vi "micro1 pvgen300.vi"(0 "FluxStrIn":string, 1 "Numin":i32, 5 "errin":errorcluster, 6 "Data label":string, 8 "tab ref":string[][](array[string]), 10 "ligne à traiter":string[](array[string])) -> (14 "result string":string, 15 "Numout":i32, 19 "errout":errorcluster)   [LabVIEW 2020]
uses:
  VG/VG_DeltaTcell.vi
  ZEN8 Semi Auto EMC/OP700/VG/VG_TCellmax.vi
  ZEN8 Semi Auto EMC/OP700/VG/VG_TCellmin.vi
  VG/IS30%.vi
  VG/VG_VCellMin70.vi
  VG/VG_VCellMax70.vi
  VG/VG_VCellMin30.vi
  VG/VG_VCellMax30.vi
  VG/VG_DeltaVcell.vi
  <vilib>/regexp/Match Regular Expression.xnode
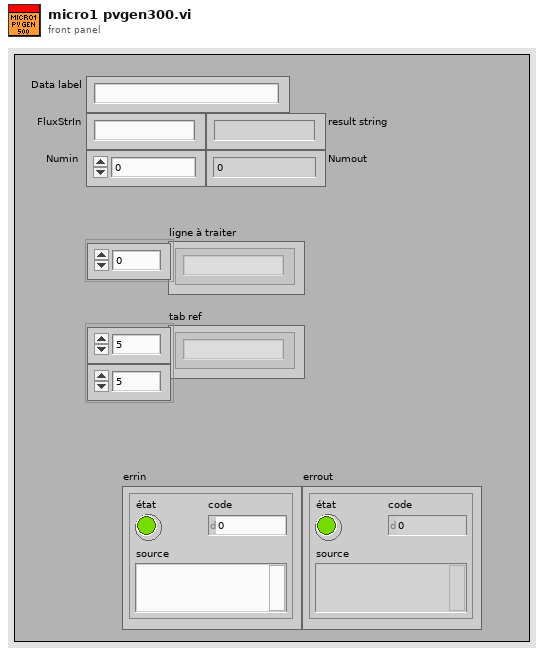
[diagram p1: front panel]
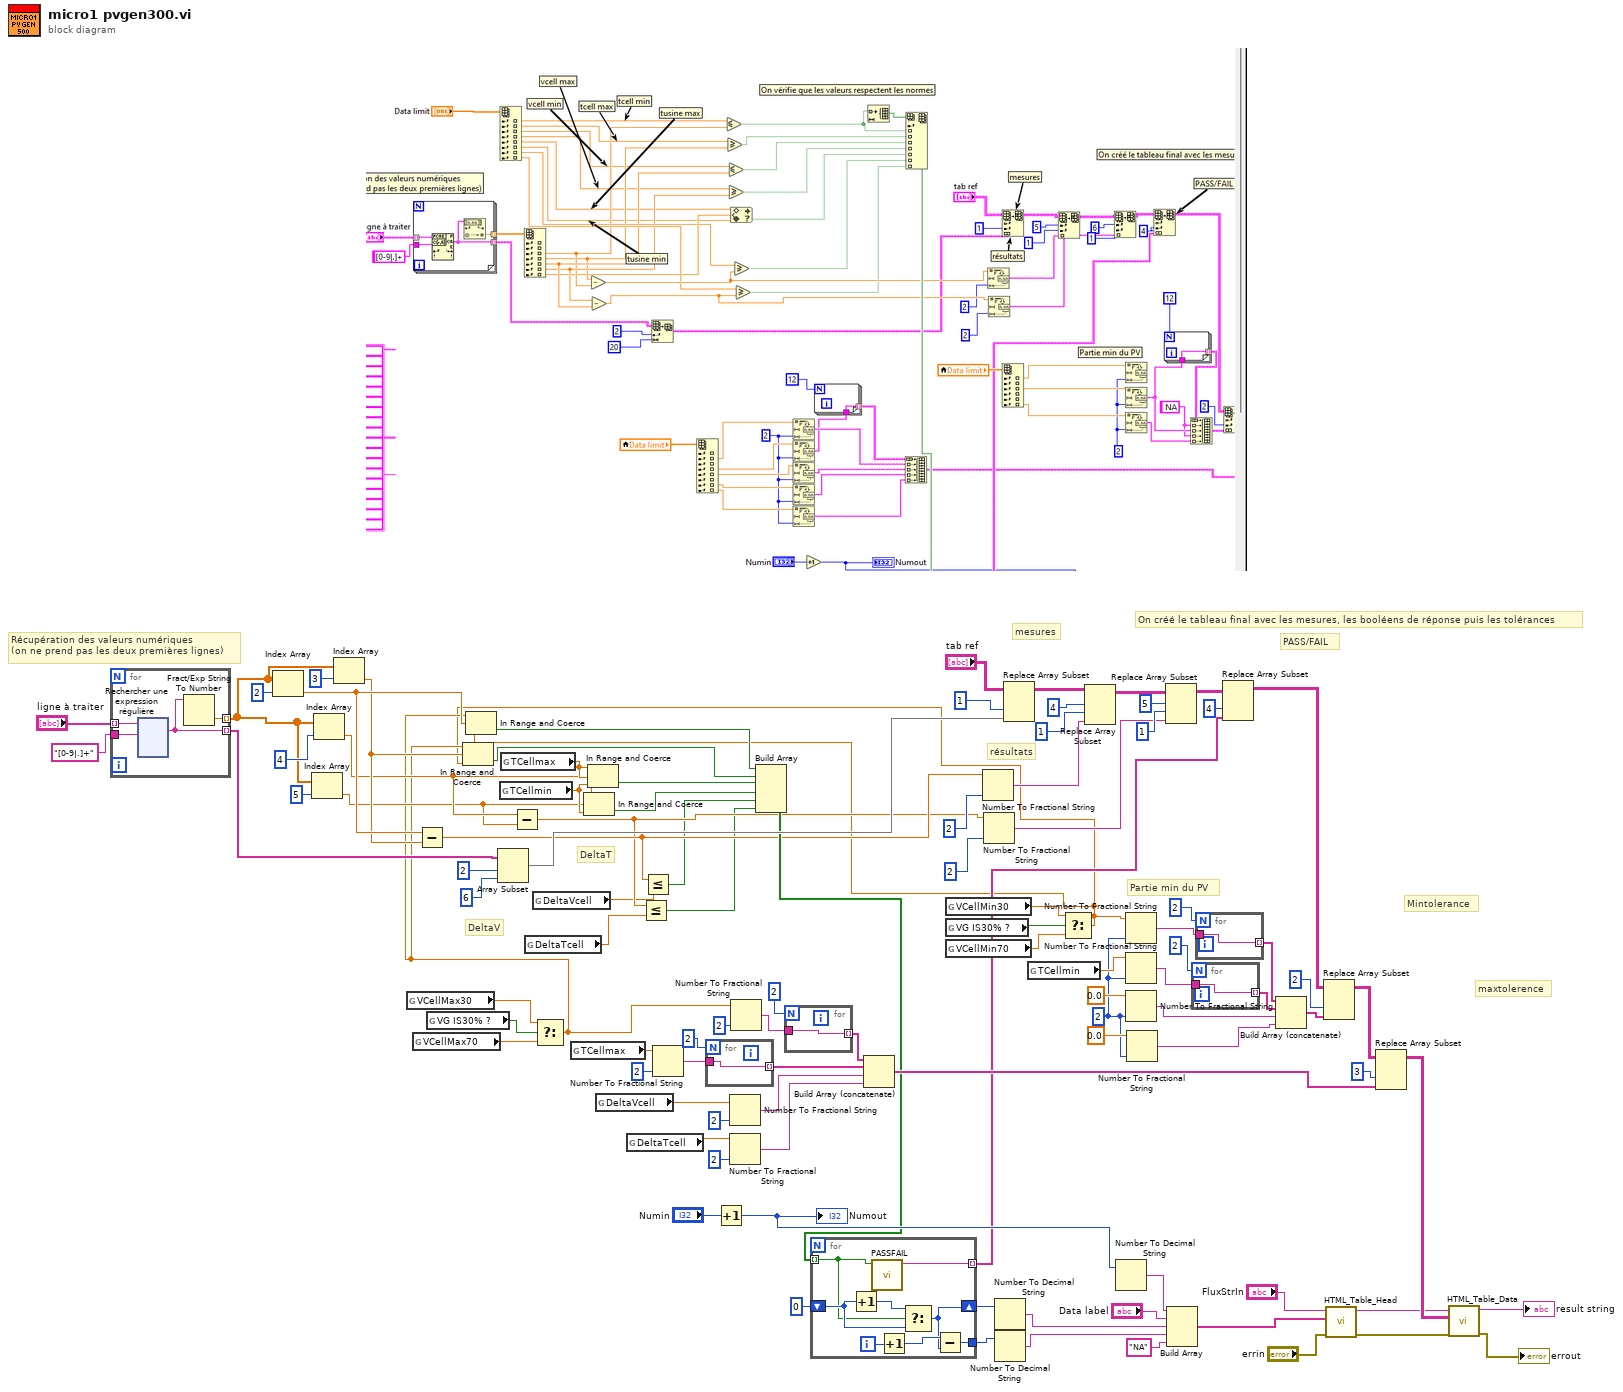
[diagram p0: block diagram]
diagram:
  w30 = 2
  # "DeltaV"
  # "DeltaT"
  # "Partie min du PV"
  # "Récupération des valeurs numériques\n(on ne prend pas les deux premières lignes)"
  # "On créé le tableau final avec les mesures, les booléens de réponse puis les tolérances"
  # "maxtolerence"
  # "Mintolerance"
  # "mesures"
  # "PASS/FAIL"
  # "résultats"
  n1 = for {
    tunnel: "ligne à traiter" -> [w106] mode=indexing
    tunnel: "[0-9|.]+" ("expression régulière") -> [w105]
    tunnel: [w104] -> w19 mode=indexing
    tunnel: [w103] -> w70 mode=indexing
    n2 = xnode "Rechercher une expression régulière"("input string"=w106, "regular expression"=w105) -> ("whole match"=w103:string)  [unwired: 4 in, 4 out]
    n3 = Fract/Exp String To Number(string=w103) -> (number=w104:dbl)  [unwired: 3 in, 1 out]
  }
  n4 = Index Array(array=w19, index=2 ("indice")) -> (element=w14:dbl)
  n5 = Index Array(array=w19, index=5 ("indice")) -> (element=w11:dbl)
  n6 = Index Array(array=w19, index=4 ("longueur")) -> (element=w12:dbl)
  n7 = Index Array(array=w19, index=3 ("indice")) -> (element=w13:dbl)
  n8 = global read "VG_VCellMax30.vi" "VCellMax30"() -> (w9:dbl)
  n9 = global read "VG_VCellMax70.vi" "VCellMax70"() -> (w8:dbl)
  n10 = Subtract(x=w14, y=w13) -> (x-y=w28:dbl)
  n11 = global read "IS30%.vi" "VG IS30% ?"() -> (w10:bool)
  n12 = Array Subset(array=w70, index=2 ("indice"), length=6 ("longueur")) -> (w73:string[])
  n13 = global read "VG_TCellmin.vi" "TCellmin"() -> (w16:dbl)
  n14 = global read "VG_TCellmax.vi" "TCellmax"() -> (w17:dbl)
  n15 = Subtract(x=w12, y=w11) -> (x-y=w26:dbl)
  n16 = global read "VG_DeltaTcell.vi" "DeltaTcell"() -> (w27:dbl)
  n17 = global read "VG_DeltaVcell.vi" "DeltaVcell"() -> (w2:dbl)
  n18 = Select(t=w9, s=w10, f=w8) -> (s? t:f=w4:dbl)
  n19 = global read "VG_TCellmax.vi" "TCellmax"() -> (w47:dbl)
  n20 = In Range and Coerce(upper limit=w17, x=w11, lower limit=w16) -> (In Range?=w15:bool)  [unwired: 1 out]
  n21 = In Range and Coerce(upper limit=w17, x=w12, lower limit=w16) -> (In Range?=w35:bool)  [unwired: 1 out]
  n22 = global read "VG_DeltaVcell.vi" "DeltaVcell"() -> (w1:dbl)
  n23 = global read "VG_DeltaTcell.vi" "DeltaTcell"() -> (w46:dbl)
  n24 = Less Or Equal?(x=w26, y=w27) -> (x <= y?=w25:bool)
  n25 = Less Or Equal?(x=w28, y=w2) -> (x <= y?=w23:bool)
  n26 = Number To Fractional String(number=w47, precision (6)=i16 2 ("précision (6)")) -> (F-format string=w43:string)  [unwired: 2 in]
  n27 = for {
    N: 2 -> [_]
    tunnel: w43 -> [w221]
    tunnel: [w221] -> w42 mode=indexing
  }
  n28 = Increment(x="Numin") -> (x+1=w88:i32)
  "Numout" <- w88
  n29 = Number To Fractional String(number=w1, precision (6)=i16 2 ("précision (6)")) -> (F-format string=w45:string)  [unwired: 2 in]
  n30 = Number To Fractional String(number=w46, precision (6)=i16 2 ("précision (6)")) -> (F-format string=w44:string)  [unwired: 2 in]
  n31 = Number To Fractional String(number=w4, precision (6)=i16 2 ("précision (6)")) -> (F-format string=w48:string)  [unwired: 2 in]
  n32 = for {
    N: 2 -> [_]
    tunnel: w48 -> [w222]
    tunnel: [w222] -> w57 mode=indexing
  }
  n33 = Build Array (concatenate)(w57, w42, w45, w44) -> (w102:string[])
  n34 = global read "VG_VCellMin30.vi" "VCellMin30"() -> (w5:dbl)
  n35 = global read "IS30%.vi" "VG IS30% ?"() -> (w7:bool)
  n36 = global read "VG_VCellMin70.vi" "VCellMin70"() -> (w6:dbl)
  n37 = Number To Fractional String(number=w28, precision (6)=i16 2) -> (F-format string=w62:string)  [unwired: 2 in]
  n38 = Number To Fractional String(number=w26, precision (6)=i16 2) -> (F-format string=w59:string)  [unwired: 2 in]
  n39 = Replace Array Subset(array="tab ref", new element=w73, index (col)=1 ("indice désactivé (col)")) -> (w66:string[][])  [unwired: 1 in]
  n40 = global read "VG_TCellmin.vi" "TCellmin"() -> (w40:dbl)
  n41 = Select(t=w5, s=w7, f=w6) -> (s? t:f=w3:dbl)
  n42 = In Range and Coerce(upper limit=w4, x=w13, lower limit=w3) -> (In Range?=w20:bool)  [unwired: 1 out]
  n43 = In Range and Coerce(upper limit=w4, x=w14, lower limit=w3) -> (In Range?=w22:bool)  [unwired: 1 out]
  n44 = Build Array(w22, w20, w35, w15, w23, w25) -> (w34:bool[])
  n45 = for {
    tunnel: w34 -> [w223] mode=indexing
    tunnel: [w224] -> w71 mode=indexing
    shift-right: [w226] -> w90
    shift-left: 0 -> [w229]
    tunnel: [w225] -> w91
    i -> [w228]
    n46 = Increment(x=w229) -> (x+1=w230:i32)
    n47 = call <userlib>:"PASSFAIL.vi"("E"=w223) -> ("S"=w224:string)  [unwired: 10 in]
    n48 = Increment(x=w228) -> (x+1=w227:i32)
    n49 = Select(t=w230, s=w223, f=w229) -> (s? t:f=w226:i32)
    n50 = Subtract(x=w227, y=w226) -> (x-y=w225:i32)
  }
  n51 = Number To Decimal String(number=w90) -> (decimal integer string=w92:string)  [unwired: 1 in]
  n52 = Number To Decimal String(number=w91) -> (decimal integer string=w93:string)  [unwired: 1 in]
  n53 = Replace Array Subset(array=w66, new element=w62, index (row)=4 ("disabled index (row)"), index (col)=1 ("disabled index (col)")) -> (w64:string[][])
  n54 = Number To Decimal String(number=w88) -> (decimal integer string=w76:string)  [unwired: 1 in]
  n55 = Number To Fractional String(number=w3, precision (6)=w30) -> (F-format string=w41:string)  [unwired: 2 in]
  n56 = Number To Fractional String(number=w40, precision (6)=w30) -> (F-format string=w33:string)  [unwired: 2 in]
  n57 = Number To Fractional String(number=0.0 ("nombre"), precision (6)=w30) -> (F-format string=w38:string)  [unwired: 2 in]
  n58 = Number To Fractional String(number=0.0 ("nombre"), precision (6)=w30) -> (F-format string=w36:string)  [unwired: 2 in]
  n59 = Replace Array Subset(array=w64, new element=w59, index (row)=5 ("disabled index (row)"), index (col)=1 ("disabled index (col)")) -> (w63:string[][])
  n60 = Build Array(w76, "Data label", w92, w93, "NA" ("élément")) -> (w79:string[])
  n61 = for {
    N: 2 -> [_]
    tunnel: w33 -> [w231]
    tunnel: [w231] -> w32 mode=indexing
  }
  n62 = for {
    N: 2 -> [_]
    tunnel: w41 -> [w232]
    tunnel: [w232] -> w54 mode=indexing
  }
  n63 = Replace Array Subset(array=w63, new element=w71, index (col)=4 ("indice désactivé (col)")) -> (w96:string[][])  [unwired: 1 in]
  n64 = Build Array (concatenate)(w54, w32, w38, w36) -> (w101:string[])
  n65 = Replace Array Subset(array=w96, new element=w101, index (col)=2 ("indice désactivé (col)")) -> (w98:string[][])  [unwired: 1 in]
  n66 = call "HTML_Table_Head.vi"("entrée d'erreur (pas d'erreur)"="errin", "Tableau"=w79, "chaîne en entrée"="FluxStrIn") -> ("sortie d'erreur"=w78:errorcluster, "result string"=w77:string)  [unwired: 7 in]
  n67 = Replace Array Subset(array=w98, new element=w102, index (col)=3 ("indice désactivé (col)")) -> (w97:string[][])  [unwired: 1 in]
  n68 = call "HTML_Table_Data.vi"("entrée d'erreur (pas d'erreur)"=w78, "Tableau"=w97, "chaîne en entrée"=w77) -> ("sortie d'erreur"=→"errout":errorcluster, "result string"=→"result string":string)  [unwired: 7 in]
